vi "Encoders.vi"(8 "error in (no error)":errorcluster) -> (0 "error out":errorcluster, 3 "Encoder Data":T1)   [LabVIEW 2014]
uses:
  <userlib>/UCSD Robotics Lab/Robotics-Cape/LV/libroboticscape.lvlib
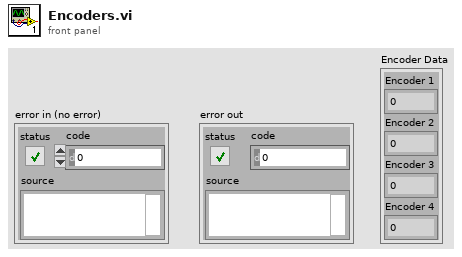
[diagram p1: front panel]
types:
  T1 = cluster{"Encoder 1":i32, "Encoder 2":i32, "Encoder 3":i32, "Encoder 4":i32}
  T2 = cluster{"function return":i32, "function return":i32, "function return":i32, "function return":i32}
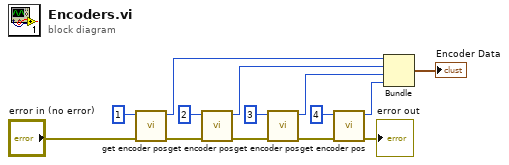
[diagram p0: block diagram]
diagram:
  n1 = call <userlib>:"get encoder pos.vi"("error in (no error)"="error in (no error)", "ch"=1) -> ("error out"=w7:errorcluster, "function return"=w5:i32)  [unwired: 8 in]
  n2 = call <userlib>:"get encoder pos.vi"("error in (no error)"=w7, "ch"=2) -> ("error out"=w8:errorcluster, "function return"=w1:i32)  [unwired: 8 in]
  n3 = call <userlib>:"get encoder pos.vi"("error in (no error)"=w8, "ch"=3) -> ("error out"=w9:errorcluster, "function return"=w4:i32)  [unwired: 8 in]
  n4 = call <userlib>:"get encoder pos.vi"("error in (no error)"=w9, "ch"=4) -> ("error out"=→"error out":errorcluster, "function return"=w3:i32)  [unwired: 8 in]
  n5 = Bundle("function return"=w5, "function return"=w1, "function return"=w4, "function return"=w3) -> (→"Encoder Data":T2)  [unwired: 1 in]
